vi "Set Verbose Level.vi"(8 "error in (no error)":errorcluster, 10 "Verbose Level":i32) -> (0 "error out":errorcluster)   [LabVIEW 2013, in "SET_Printf.lvlib" / "LV_Printf Core.lvclass"]
uses:
  LV_Printf Core.lvclass
  LV_Printf Core.lvclass/LV_Printf Core.ctl
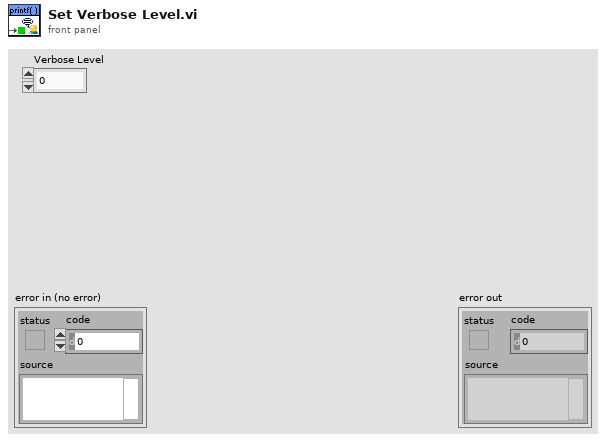
[diagram p1: front panel]
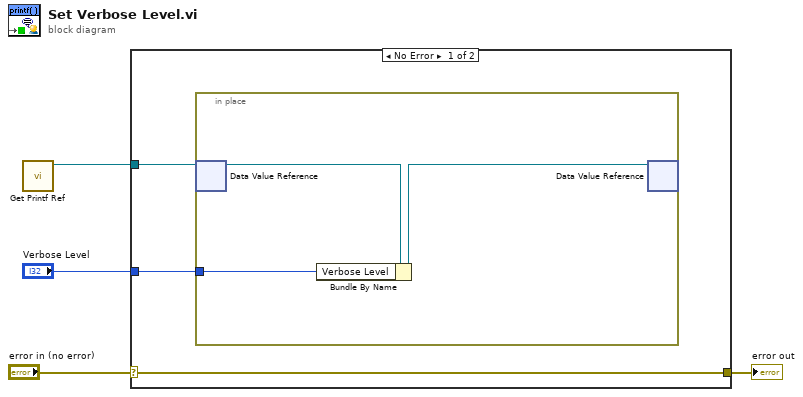
[diagram p0: block diagram]
diagram:
  n1 = call "Get Printf Ref.vi"() -> ("Printf DVR"=w2:refnum<data-value>)  [unwired: 11 in]
  n2 = case shown="No Error" "error in (no error)" {
    selector: "error in (no error)" -> [w7 w11]
    tunnel: [w7 w11] -> w3
    tunnel: w2 -> [w6 _]
    tunnel: "Verbose Level" -> [w5 _]
    frame No Error {
      n3 = in-place {
        in-place-border: w5 -> [w8]
        n4 = in-place-dvr #1(w6) -> (w10:refnum<class "LV_Printf Core.lvclass">)  [unwired: 1 out]
        n5 = Bundle By Name(cluster=w10, "Verbose Level"=w8) -> (w9:refnum<class "LV_Printf Core.lvclass">)
        n6 = in-place-dvr #1(w9) -> ()  [unwired: 2 out]
      }
    }
    frame Error {
    }
  }
  "error out" <- w3
